vi "mlink_disconnect.vi"(8 "error in (no error)":errorcluster, 11 "connection ID":i32=-1) -> (0 "error out":errorcluster)   [LabVIEW 2009, in "MicroDAQ.lvlib" / "mlink.lvlib"]
doc: "This function closes connection with MicroDAQ."
uses:
  <instrlib>/MicroDAQ/Mlink library wraper/mlink.lvlib
  <instrlib>/MicroDAQ/MLink32.dll
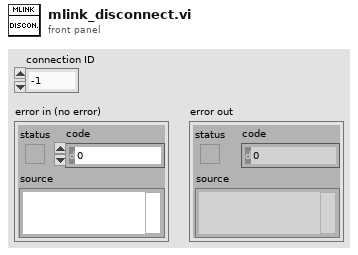
[diagram p1: front panel]
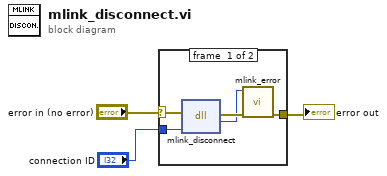
[diagram p0: block diagram]
diagram:
  n1 = case shown="No Error" "error in (no error)" {
    selector: "error in (no error)" -> [w7 w9]
    tunnel: "connection ID" -> [w8 _]
    tunnel: [w5 w9] -> w1
    frame #0 {
      n2 = dll-call lib="C:/Program Files (x86)/National Instruments/LabVIEW 2009/instr.lib/MicroDAQ/MLink32.dll" fn="mlink_disconnect"(error in=w7, "connection ID"=w8) -> (error out=w6:errorcluster, "return type"=w4:i32)  [unwired: 3 in, 1 out]
      n3 = call <instrlib>:"mlink_error.vi"("error in (no error)"=w6, "error code"=w4) -> ("error out"=w5:errorcluster)  [unwired: 9 in]
    }
    frame #1 {
    }
  }
  "error out" <- w1
